vi "2000511 labview.vi"() -> ()   [LabVIEW 2017]
panel:
  out "Gauge":dbl(knob) scale=0.0..10.0
  in  "Array":void[](array[numeric])
  in  "Numeric Control":dbl
  out "Boolean 2":bool
  in  "Boolean":bool
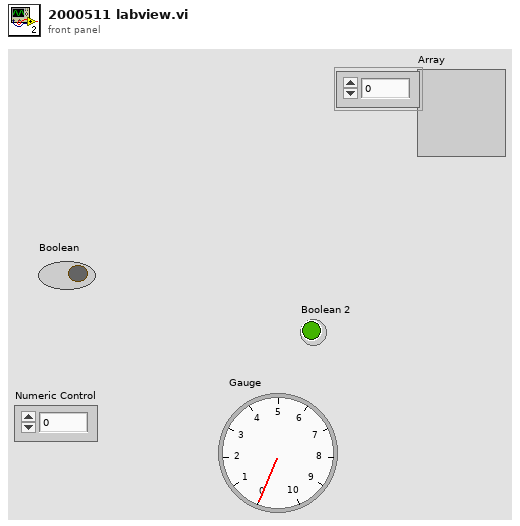
[diagram p1: front panel]
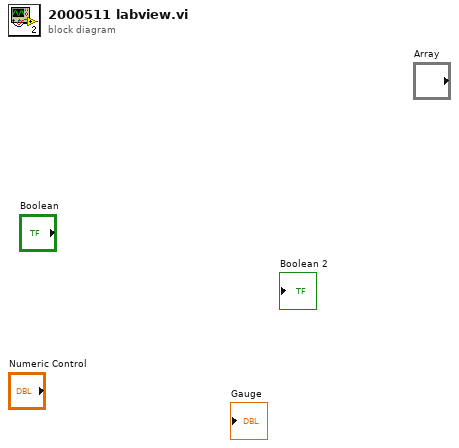
[diagram p0: block diagram]
diagram:
